vi "Write Element of In State.vi"(8 "error in (no error)":errorcluster, 9 "in state":bool, 10 "index":i32, 11 "CS++DCPwrChannelData in":refnum<class "CS++DCPwrChannelData.lvclass">) -> (0 "error out":errorcluster, 3 "CS++DCPwrChannelData out":refnum<class "CS++DCPwrChannelData.lvclass">)   [LabVIEW 2015, in "CS++DCPwrGui.lvlib" / "CS++DCPwrChannelData.lvclass"]
uses:
  CS++DCPwrChannelData.lvclass
  CS++DCPwrChannelData.lvclass/CS++DCPwrChannelData.ctl
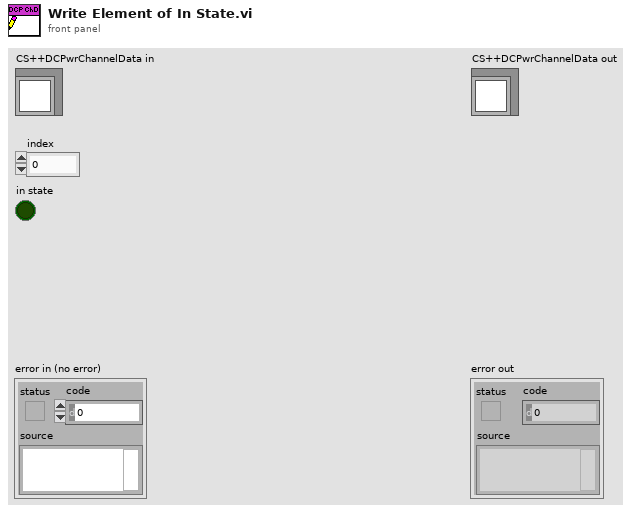
[diagram p1: front panel]
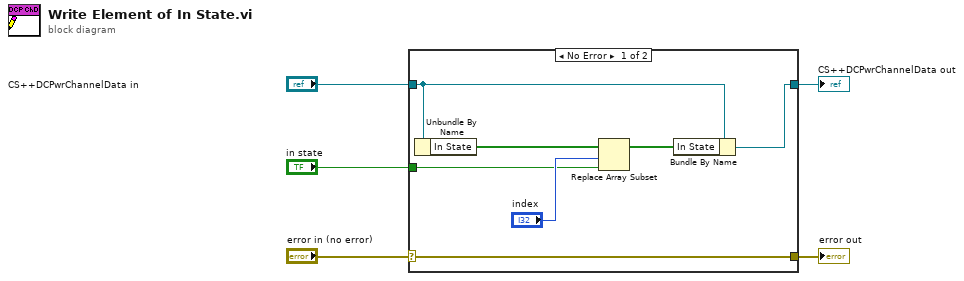
[diagram p0: block diagram]
diagram:
  n1 = case shown="No Error" "error in (no error)" {
    selector: "error in (no error)" -> [w12 w13]
    tunnel: [w12 w13] -> w4
    tunnel: [w11 w14] -> w2
    tunnel: "CS++DCPwrChannelData in" -> [w10 w14]
    tunnel: "in state" -> [w6 _]
    frame No Error {
      n2 = Unbundle By Name(w10) -> ("In State"=w9:bool[])
      n3 = Replace Array Subset(array=w9, new element=w6, index="index") -> (w8:bool[])
      n4 = Bundle By Name(cluster=w10, "In State"=w8) -> (w11:refnum<class "CS++DCPwrChannelData.lvclass">)
    }
    frame Error {
    }
  }
  "error out" <- w4
  "CS++DCPwrChannelData out" <- w2
